vi "Logfile.vi"   [LabVIEW 2011]
uses:
  _GlobalVariables&Libraries/ATV Program Global Variables.vi
  <vilib>/Utility/file.llb/Write To Spreadsheet File (DBL).vi
types:
  T1 = cluster{"End ATV Program":bool, "E-Stop":bool, "Save Logfile":bool, "Logfile Iteration Delay \n(milliseconds)":u32}
  T2 = cluster{"GPS VISA resource name":refnum<visa-resource-name>, "GPS Error":errorcluster, "Disable GPS VISA":bool, "Latitude":dbl, "Longitude":dbl}
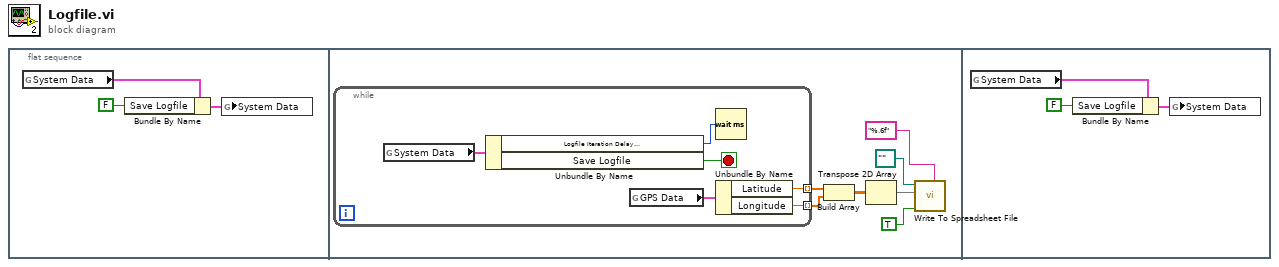
[diagram p0: block diagram]
diagram:
  n1 = flat-sequence {
    frame #0 {
      n2 = global read "ATV Program Global Variables.vi" "System Data"() -> (w3:T1)
      n3 = Bundle By Name(cluster=w3, "Save Logfile"=FALSE) -> (w2:T1)
      n4 = global write "ATV Program Global Variables.vi" "System Data"(w2) -> ()
    }
    frame #1 {
      n5 = while {
        tunnel: [w12] -> w10 mode=indexing
        tunnel: [w11] -> w9 mode=indexing
        stop <- w15 stop-if-true
        n6 = global read "ATV Program Global Variables.vi" "System Data"() -> (w16:T1)
        n7 = Unbundle By Name(w16) -> ("Logfile Iteration Delay \n(milliseconds)"=w14:u32, "Save Logfile"=w15:bool)
        n8 = global read "ATV Program Global Variables.vi" "GPS Data"() -> (w13:T2)
        n9 = Wait (ms)(milliseconds to wait=w14) -> ()  [unwired: 1 out]
        n10 = Unbundle By Name(w13) -> ("Latitude"=w12:dbl, "Longitude"=w11:dbl)
      }
      n11 = Build Array(w10, w9) -> (w8:dbl[][])
      n12 = Transpose 2D Array(2D array=w8) -> (transposed array=w7:dbl[][])
      n13 = call-poly <vilib>:"Write To Spreadsheet File.vi"("format (%.3f)"="%.6f", "append to file? (new file:F)"=TRUE, "2D data"=w7, "file path (dialog if empty)"=path "") -> ()  [unwired: 4 in, 1 out]
    }
    frame #2 {
      n14 = global read "ATV Program Global Variables.vi" "System Data"() -> (w17:T1)
      n15 = Bundle By Name(cluster=w17, "Save Logfile"=FALSE) -> (w18:T1)
      n16 = global write "ATV Program Global Variables.vi" "System Data"(w18) -> ()
    }
  }
